vi "Rohde & Schwarz VNA Read Trigger Mode.vi"(6 "Channel":i8=1 min=1 max=99 step=1, 7 "Rohde & Schwarz VNA":T1, 8 "error in (no error)":errorcluster, 11 "VISA Resource Name":refnum<visa-resource-name>) -> (0 "error out":errorcluster, 2 "Trigger Mode":T2, 3 "dup VISA Resource Name":refnum<visa-resource-name>)   [LabVIEW 2011]
doc: "This VI for the HP8753B Network Analyzers reads the stimulus values. Except when performing log sweeps and freq list sweeps, this VI uses the start and stop values and the number of points to calcuate the stimulus values."
uses:
  TypeDefs/Rohde & Schwarz VNA Trigger Mode.ctl
  TypeDefs/Rohde & Schwarz VNA Instrument Info.ctl
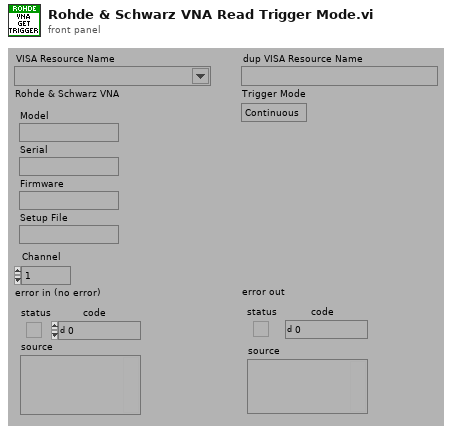
[diagram p1: front panel]
types:
  T1 = typedef "Rohde & Schwarz VNA Instrument Info.ctl" = cluster{"Model":string, "Serial":string, "Firmware":string, "Setup File":string}
  T2 = typedef "Rohde & Schwarz VNA Trigger Mode.ctl" = enum16{"Continuous", "Hold", "Single"}
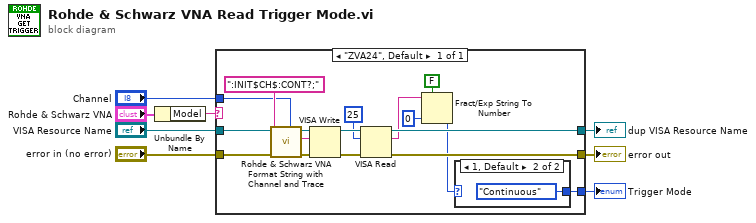
[diagram p0: block diagram]
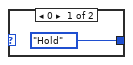
[diagram p2: hidden frame]
diagram:
  n1 = Unbundle By Name("Rohde & Schwarz VNA") -> ("Model"=w1:string)
  n2 = case shown="\"ZVA24\", Default" w1 {
    tunnel: "error in (no error)" -> [w23]
    tunnel: [w21] -> w7
    tunnel: "VISA Resource Name" -> [w18]
    tunnel: [w20] -> w5
    tunnel: [w12] -> w4
    tunnel: "Channel" -> [w9]
    frame "ZVA24", Default {
      n3 = call "Rohde & Schwarz VNA Format String with Channel and Trace.vi"("Trace"=w9, "String"=":INIT$CH$:CONT?;") -> ("String Out"=w10:string)  [unwired: 1 in, 6 out]
      n4 = VISA Write(VISA resource name=w18, write buffer=w10, error in (no error)=w23) -> (VISA resource name out=w19:refnum<visa-resource-name>, error out=w22:errorcluster)  [unwired: 1 out]
      n5 = VISA Read(VISA resource name=w19, byte count=u32 25, error in (no error)=w22) -> (VISA resource name out=w20:refnum<visa-resource-name>, read buffer=w15:string, error out=w21:errorcluster)  [unwired: 1 out]
      n6 = Fract/Exp String To Number(use system decimal point (T)=FALSE, string=w15, default (0 dbl)=0 ("default (0 DBL)")) -> (number=w13:i32)  [unwired: 2 out]
      n7 = case shown="1, Default" w13 {
        tunnel: [Rohde_&_Schwarz_VNA_Trigger_Mode."Hold" Rohde_&_Schwarz_VNA_Trigger_Mode."Continuous"] -> w12
        frame 0 {
        }
        frame 1, Default {
        }
      }
    }
  }
  "dup VISA Resource Name" <- w5
  "error out" <- w7
  "Trigger Mode" <- w4
